vi "Monitoring Page.vi"(8 "error in (no error)":errorcluster, 11 "Node Ptr":T1 format="%.0x") -> (0 "error out":errorcluster)   [LabVIEW 2017, in "DSF System Explorer.lvlib"]
uses:
  DSF System Explorer.lvlib
  <vilib>/NI Veristand/Custom Device API/Custom Device Item Ref.ctl
  <vilib>/NI Veristand/Custom Device API/Custom Device API.lvlib
panel:
  in  "Header":cluster{"Section Name":string}={"Section Name"="Monitoring"}
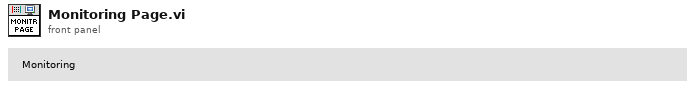
[diagram p1: front panel]
types:
  T1 = typedef "Custom Device API.lvlib/Custom Device Item Ref.ctl" = u64
  T2 = typedef "Custom Device API.lvlib/Custom Device Commands.ctl" = enum16{"Default", "Item renamed", "Shutdown", "Dynamic button pressed"}
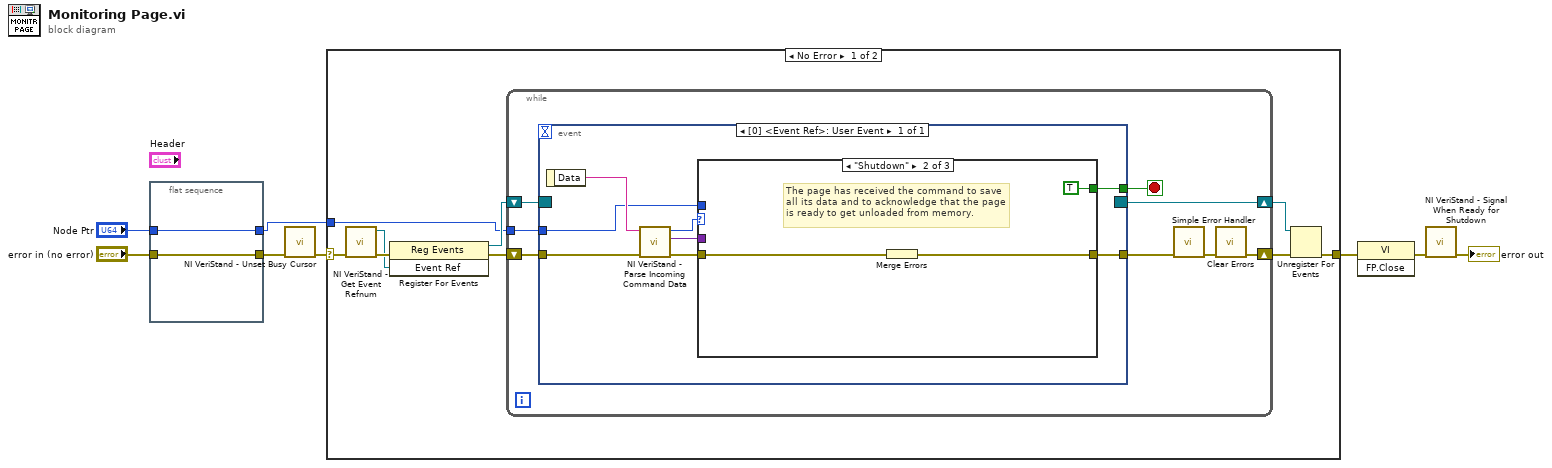
[diagram p0: block diagram]
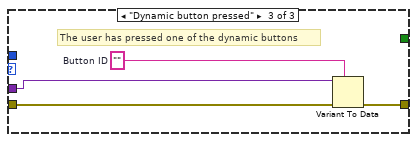
[diagram p3: hidden frame]
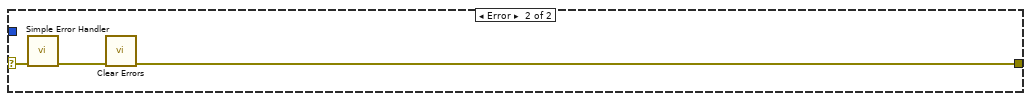
[diagram p4: hidden frame]
diagram:
  n1 = flat-sequence "Initialization code" {
    tunnel: "error in (no error)" -> [w9]
    tunnel: "Node Ptr" -> [w10]
    tunnel: [w9] -> w4
    tunnel: [w10] -> w1
    frame #0 {
    }
  }
  n2 = call <vilib>:"NI VeriStand - Unset Busy Cursor.vi"("error in (no error)"=w4) -> ("error out"=w3:errorcluster)  [unwired: 10 out]
  n3 = case shown="No Error" w3 {
    selector: w3 -> [w11 w46]
    tunnel: [w16 w44] -> w8
    tunnel: w1 -> [w12 _]
    frame No Error {
      n4 = call <vilib>:"NI VeriStand - Get Event Refnum.vi"("error in (no error)"=w11) -> ("error out"=w19:errorcluster, "Event Ref"=w15:refnum<user-event>)  [unwired: 9 out]
      n5 = register-events(error in=w19, w15) -> (reference out=w13:refnum<event-registration>, error out=w14:errorcluster)  [unwired: 1 in]
      n6 = while {
        tunnel: w12 -> [w23]
        shift-right: [w20] -> w17
        shift-left: w14 -> [w26]
        shift-right: [w27] -> w18
        shift-left: w13 -> [w25]
        stop <- w24 stop-if-true
        n7 = event shown="[0] <Event Ref>: User Event" {
          selector: w25 -> [_]
          dyn-events: [_] -> w27
          timeout: _ -> [_]
          tunnel: w26 -> [w35]
          tunnel: [w31] -> w24
          tunnel: [w30] -> w22
          tunnel: w23 -> [w29]
          event User Event {
            n8 = event-data() -> ("Data"=w34:string)  [unwired: 1 out]
            n9 = call <vilib>:"NI VeriStand - Parse Incoming Command Data.vi"("error in (no error)"=w35, "Incoming data"=w34) -> ("error out"=w33:errorcluster, "Outgoing data"=w28:variant, "Action"=w32:T2)  [unwired: 7 out]
            n10 = case shown="\"Shutdown\"" w32 {
              tunnel: w33 -> [w36 w38 w43]
              tunnel: [_ TRUE _] -> w31
              tunnel: [w36 w37 w40] -> w30
              tunnel: w29 -> [_ _ _]
              tunnel: w28 -> [_ _ w42]
              frame "Default", Default {
              }
              frame "Shutdown" {
                # "The page has received the command to save all its data and to acknowledge that the page is ready to get unloaded from memory."
                n11 = Merge Errors(w38) -> (w37:errorcluster)
              }
              frame "Dynamic button pressed" {
                w41 = ""  # Button ID
                # "The user has pressed one of the dynamic buttons"
                n12 = Variant To Data(error in=w43, type=w41, Variant=w42) -> (error out=w40:errorcluster)  [unwired: 1 out]
              }
            }
          }
        }
        n13 = call <vilib>:"Simple Error Handler.vi"("error in (no error)"=w22) -> ("error out"=w21:errorcluster)  [unwired: 1 in, 7 out]
        n14 = call <vilib>:"Clear Errors.vi"("error in (no error)"=w21) -> ("error out"=w20:errorcluster)  [unwired: 1 in, 5 out]
      }
      n15 = Unregister For Events(event registration refnum=w18, error in=w17) -> (error out=w16:errorcluster)
    }
    frame Error {
      n16 = call <vilib>:"Simple Error Handler.vi"("error in (no error)"=w46) -> ("error out"=w45:errorcluster)  [unwired: 1 in, 7 out]
      n17 = call <vilib>:"Clear Errors.vi"("error in (no error)"=w45) -> ("error out"=w44:errorcluster)  [unwired: 1 in, 5 out]
    }
  }
  n18 = invoke class="VI" method="FP.Close"(error in=w8) -> (error out=w7:errorcluster)  [unwired: 2 in, 2 out]
  n19 = call <vilib>:"NI VeriStand - Signal When Ready for Shutdown.vi"("error in (no error)"=w7) -> ("error out"=→"error out":errorcluster)  [unwired: 10 out]
